vi "_PC_Pub_ReadRTScript.vi"(8 "error in (no error)":errorcluster) -> (0 "error out":errorcluster, 2 "script string":string)   [LabVIEW 2018]
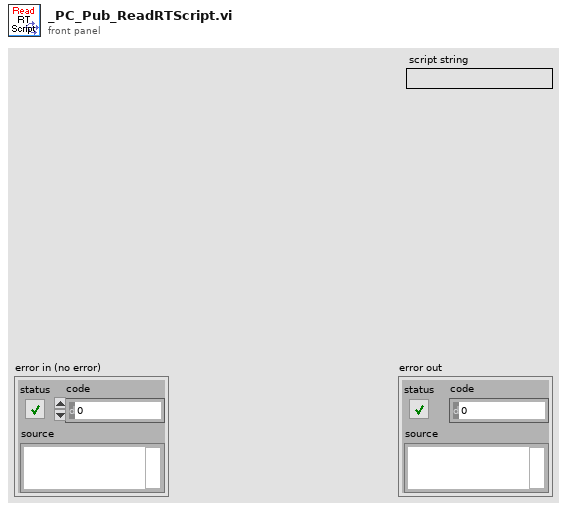
[diagram p1: front panel]
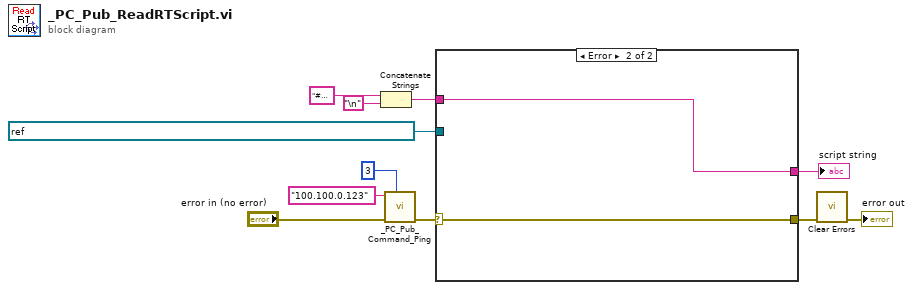
[diagram p0: block diagram]
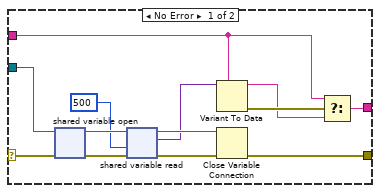
[diagram p2: hidden frame]
diagram:
  n1 = Concatenate Strings("#Header(IonTrap.R0=10,IonTrap.Z0=7.07106781187, MaxAmp=330);\nUpdConj:: IniPhase=2147483648, PhaseDiff=2147483648 2147483648, ConjLen=0 0, FixedLen=F;\nSetDAQ::Channel=0,SampRate=0;\nStart:: Freq=200000, Amp=200, WfmType=0;\nStop::;\n" ("Script of MS Process"), "\n") -> (w5:string)
  n2 = call "_PC_Pub_Command_Ping.vi"("Loop Times"=3, "error in (no error)"="error in (no error)", "PCIP String"="100.100.0.123") -> ("error out"=w8:errorcluster)  [unwired: 8 in]
  n3 = case shown="Error" w8 {
    selector: w8 -> [w22 w26]
    tunnel: refnum<k21> "ni.var.psp://NI-sbRIO/_RT_CtrlLoop_WfmData_Variable/Wfm_Script" ("shared variable refnum in") -> [w24 _]
    tunnel: [w23 w26] -> w3
    tunnel: w5 -> [w14 w25]
    tunnel: [w12 w25] -> w4
    frame No Error {
      n4 = shared-variable-open(w24, w22) -> (w21:refnum<k21>, w19:errorcluster)
      n5 = shared-variable-read(w21, w19, 500 ("timeout ms")) -> (w20:refnum<k21>, w18:errorcluster, w16:variant)  [unwired: 1 out]
      n6 = Variant To Data(type=w14, Variant=w16) -> (data=w13:string, error out=w15:errorcluster)  [unwired: 1 in]
      n7 = Close Variable Connection(8:w18, 11:w20) -> (0:w23:errorcluster)
      n8 = Select(t=w14, s=w15, f=w13) -> (s? t:f=w12:string)
    }
    frame Error {
    }
  }
  "script string" <- w4
  n9 = call <vilib>:"Clear Errors.vi"("error in (no error)"=w3) -> ("error out"=→"error out":errorcluster)  [unwired: 5 in, 1 out]
